vi "Remote Video livestream (TCP SERVER).vi"(1 "Quality":i32=750 min=0 max=1000, 2 "TCP/IP port":u16=80, 3 "Camera":T1="Travcam") -> (0 "Error out":errorcluster)   [LabVIEW 2015]
uses:
  Camera enum/Camera enum.ctl
  Globals/CamServer global.vi
panel:
  # "PN 27/08/15"
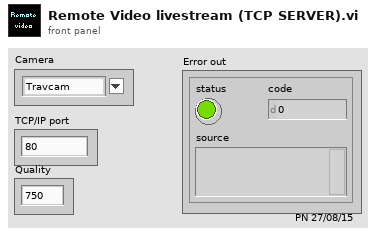
[diagram p1: front panel]
types:
  T1 = typedef "Camera enum.ctl" = string
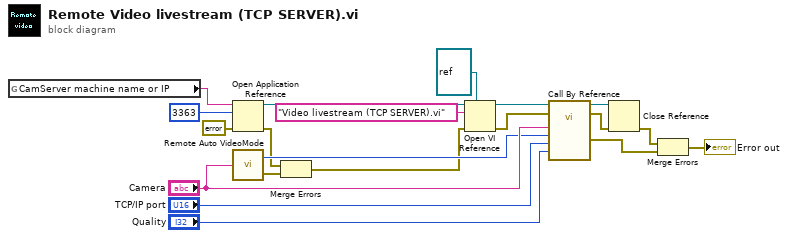
[diagram p0: block diagram]
diagram:
  n1 = global read "CamServer global.vi" "CamServer machine name or IP"() -> (w6:string)
  n2 = Open Application Reference(8:errorcluster {"status"=FALSE, "code"=0, "source"=""} ("error in (no error)"), 10:u16 3363 ("port"), 11:w6) -> (0:w3:errorcluster, 3:w18:refnum<vi>)  [unwired: 1 in]
  n3 = call "Remote Auto VideoMode.vi"("Camera"="Camera") -> ("VideoMode"=w9:u32, "Error out"=w4:errorcluster)
  n4 = Merge Errors(w3, w4) -> (w2:errorcluster)
  n5 = Open VI Reference(type specifier VI Refnum (for type only)=refnum<vi> refnum, application reference (local)=w18, vi path="Video livestream (TCP SERVER).vi" ("machine name"), error in (no error)=w2) -> (vi reference=w16:refnum<vi>, error out=w17:errorcluster)  [unwired: 2 in]
  n6 = call-by-ref "?"(reference=w16, error in=w17, "Quality"="Quality", "TCP/IP port"="TCP/IP port", "VideoMode"=w9, "Interface name"="Camera") -> (reference out=w15:refnum<vi>, error out=w14:errorcluster, "Error Out"=w13:errorcluster)
  n7 = Close Reference(reference=w15, error in (no error)=w14) -> (error out=w12:errorcluster)
  n8 = Merge Errors(w12, w13) -> (→"Error out":errorcluster)
